vi "Fire-Abort.vi"(8 "Engine Arm":bool, 10 "Abort":bool, 11 "Fire":bool) -> (0 "Solenoids":bool[](array[boolean]), 2 "Shutdown":bool, 3 "Firing":bool)   [LabVIEW 2016]
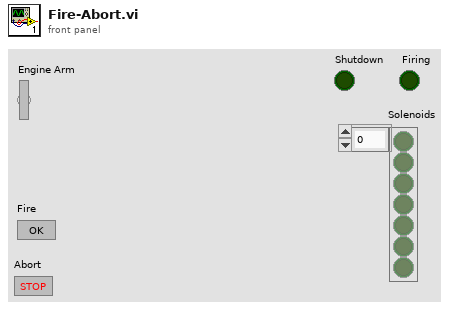
[diagram p1: front panel]
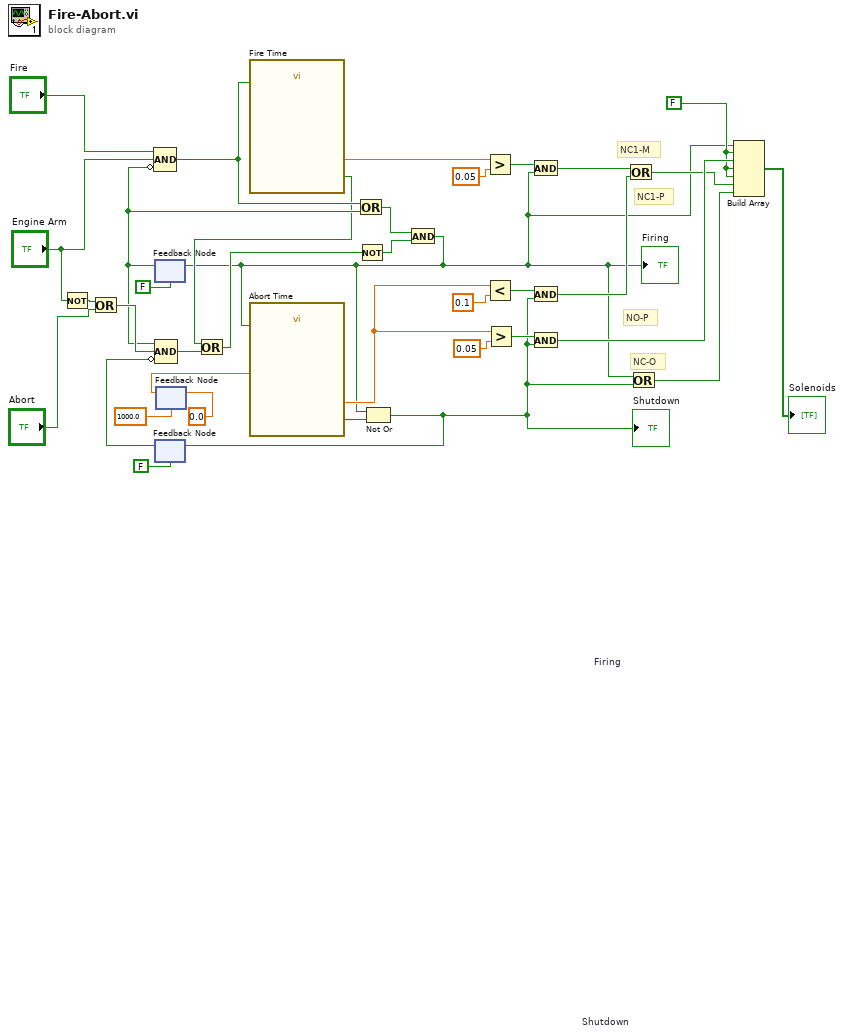
[diagram p0: block diagram]
diagram:
  w5 = FALSE
  # "NO-P"
  # "NC1-P"
  # "NC-O"
  # "NC1-M"
  n1 = Not(x="Engine Arm") -> (.not. x?=w30:bool)
  n2 = Or(x=w30, y="Abort") -> (x .or. y?=w33:bool)
  n3 = feedback #1 "Firing"(FALSE) -> (w26:bool)
  n4 = Compound Arithmetic op=AND("Fire", "Engine Arm", invert w26) -> (w23:bool)
  n5 = feedback #2 "Shutdown"(FALSE) -> (w27:bool)
  n6 = Compound Arithmetic op=AND(w26, w33, invert w27) -> (w25:bool)
  n7 = feedback #3(1000.0) -> (w1:dbl)
  n8 = feedback-in #3(0.0) -> ()
  n9 = call "Fire Time"("Reset"=w23) -> ("Elapsed Time (s)"=w20:dbl, "Time has Elapsed"=w22:bool)  [unwired: 11 in, 6 out]
  n10 = Or(x=w22, y=w25) -> (x .or. y?=w24:bool)
  n11 = Or(x=w23, y=w26) -> (x .or. y?=w29:bool)
  n12 = Not(x=w24) -> (.not. x?=w28:bool)
  n13 = And(x=w29, y=w28) -> (x .and. y?=w4:bool)
  "Firing" <- w4
  n14 = feedback-in #1(w4) -> ()
  n15 = call "Abort Time"("Reset"=w4, "Set Start Time (s)"=w1) -> ("Elapsed Time (s)"=w16:dbl, "Time has Elapsed"=w21:bool)  [unwired: 10 in, 6 out]
  n16 = Not Or(1:w21, 2:w4) -> (0:w10:bool)
  "Shutdown" <- w10
  n17 = feedback-in #2(w10) -> ()
  n18 = Greater?(x=w20, y=0.05) -> (0:w15:bool)
  n19 = Less?(x=w16, y=0.1) -> (x < y?=w14:bool)
  n20 = Greater?(x=w16, y=0.05) -> (0:w13:bool)
  n21 = And(x=w15, y=w4) -> (x .and. y?=w12:bool)
  n22 = And(x=w14, y=w10) -> (x .and. y?=w11:bool)
  n23 = And(x=w13, y=w10) -> (x .and. y?=w9:bool)
  n24 = Or(x=w12, y=w11) -> (x .or. y?=w6:bool)
  n25 = Or(x=w4, y=w10) -> (x .or. y?=w7:bool)
  n26 = Build Array(w4, w5, w9, w5, w5, w6, w7) -> (→"Solenoids":bool[])
